vi "load target.vi"(8 "error in (no error)":errorcluster, 9 "target alias":string, 11 "file path":path) -> (0 "error out":errorcluster, 3 "targets cluster out":T1)   [LabVIEW 2014, in "PL_Target Runtime.lvclass"]
uses:
  PL_Target Runtime.lvclass
  platypus configuration/targets cluster.ctl
  target configuration/PL_Target Configuration.lvclass
  platypus configuration/engines cluster.ctl
  <vilib>/NI/Module Execution Interface/Engine Configuration/engine configuration.lvclass
  <vilib>/NI/Tag Bus Module Framework/module configuration/TBM module configuration.lvclass
  <vilib>/NI/Configuration Framework/tree serializer/NISE_CEF_TreeSerializer.lvlib
  flattened data interface/PL_Serialization Interface.lvlib
  platypus configuration/PLConfigurationSerializer.lvlib
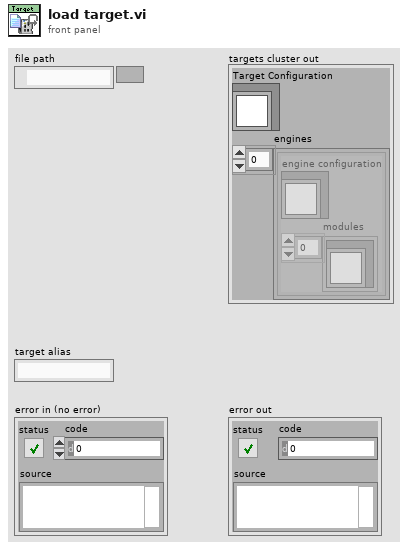
[diagram p1: front panel]
types:
  T1 = typedef "PLConfigurationSerializer.lvlib/targets cluster.ctl" = cluster{"Target Configuration":refnum<class "PL_Target Configuration.lvclass">, "engines":T2[]}
  T2 = typedef "PLConfigurationSerializer.lvlib/engines cluster.ctl" = cluster{"engine configuration":refnum<class "engine configuration.lvclass">, "modules":refnum<class "TBM module configuration.lvclass">[]}
  T3 = typedef "NISE_CEF_TreeSerializer.lvlib/base file format.ctl" = cluster{"version":string, "data":string}
  T4 = typedef "NISE_CEF_TreeSerializer.lvlib/flat hierarchy.ctl" = cluster{"hierarchy structure":T5, "instance data":T7[]}
  T5 = typedef "NISE_CEF_TreeSerializer.lvlib/full hierarchy.ctl" = cluster{"root":string, "hierarchy":T6[]}
  T6 = typedef "NISE_CEF_TreeSerializer.lvlib/hierarchy element.ctl" = cluster{"current node":string, "children":string[]}
  T7 = typedef "NISE_CEF_TreeSerializer.lvlib/instance data.ctl" = cluster{"ID":string, "Alias":string, "class":string, "version":string, "data":string}
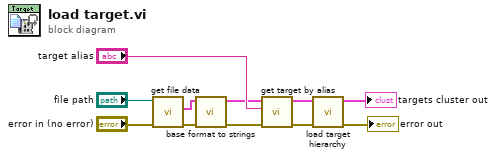
[diagram p0: block diagram]
diagram:
  n1 = call <vilib>:"get file data.vi"("error in"="error in (no error)", "Path"="file path") -> ("error out"=w3:errorcluster, "format"=w2:T3)  [unwired: 8 in]
  n2 = call <vilib>:"base format to strings.vi"("error in"=w3, "format"=w2) -> ("error out"=w6:errorcluster, "data"=w5:T4)  [unwired: 8 in]
  n3 = call "get target by alias.vi"("error in"=w6, "alias"="target alias", "system hierarchy"=w5) -> ("error out"=w9:errorcluster, "target hierarchy"=w8:T4)  [unwired: 7 in]
  n4 = call "load target hierarchy.vi"("error in"=w9, "target hierarchy"=w8) -> ("error out"=→"error out":errorcluster, "targets cluster out"=→"targets cluster out":T1)  [unwired: 8 in]
